vi "Force By Wire.vi"(8 "error in (no error)":errorcluster, 11 "Carya Config in":refnum<class "Carya Config.lvclass">) -> (0 "error out":errorcluster, 2 "Carya Config out":refnum<class "Carya Config.lvclass">, 3 "Carya Config out":refnum<class "Carya Config.lvclass">)   [LabVIEW 2013, in "Carya Config.lvclass"]
doc: "Copyright 2018, Carya Automatisering, Wiebe Walstra."
uses:
  Carya Config.lvclass
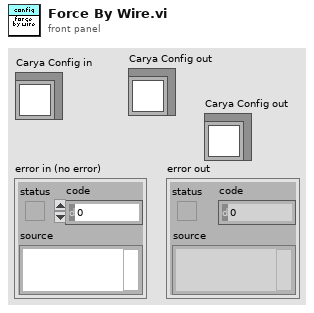
[diagram p1: front panel]
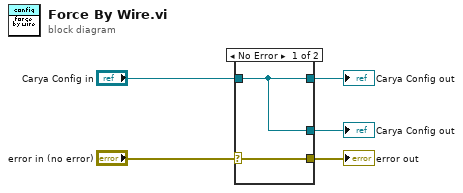
[diagram p0: block diagram]
diagram:
  n1 = case shown="No Error" "error in (no error)" {
    selector: "error in (no error)" -> [w7 w9]
    tunnel: [w7 w9] -> w4
    tunnel: [w6 w8] -> w2
    tunnel: "Carya Config in" -> [w6 w8]
    tunnel: [w6 _] -> w1
    frame No Error {
    }
    frame Error {
    }
  }
  "error out" <- w4
  "Carya Config out" <- w1
  "Carya Config out" <- w2
